vi "map_index.vi"() -> ()   [LabVIEW 2015]
panel:
  in  "index_map":u32=1
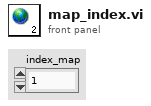
[diagram p1: front panel]
diagram:
